vi "GetCustomDeviceTimingSourceVIs.vi"(8 "error in (no error)":errorcluster, 11 "custom device reference in":refnum<k39>) -> (0 "error out":errorcluster, 2 "timing source VIs":T1(array[cluster]), 3 "custom device reference out":refnum<k39>)   [LabVIEW 2027, in "VeriStandTestUtilities.lvlib"]
uses:
  VeriStandTestUtilities.lvlib
  C:/NetCoreDLL/NationalInstruments.VeriStand.XMLReader.dll
  NetCoreDLL/NationalInstruments.VeriStand.XMLReader.dll
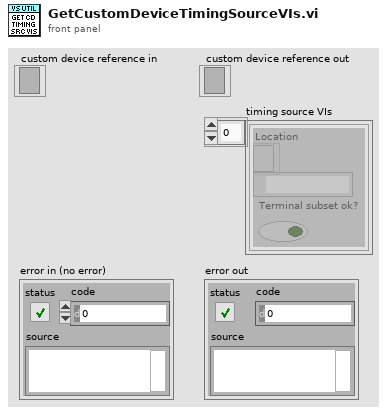
[diagram p1: front panel]
types:
  T1 = cluster{"Location":refnum<k39>, path, "Terminal subset ok?":bool}[]
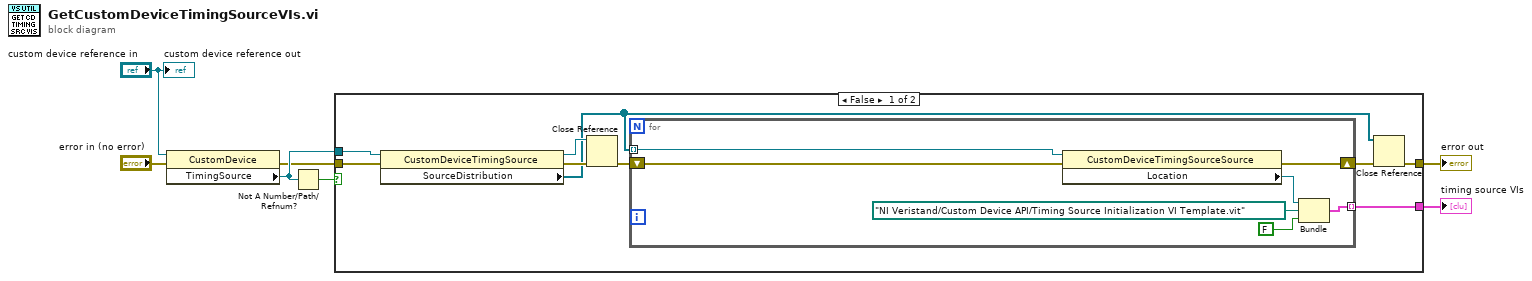
[diagram p0: block diagram]
diagram:
  n1 = property class="CustomDevice"(reference="custom device reference in", error in="error in (no error)") -> (error out=w2:errorcluster, "TimingSource"=w4:refnum<k39>)  [unwired: 1 out]
  n2 = Not A Number/Path/Refnum?(number/path/refnum=w4) -> (NaN/Path/Refnum?=w5:bool)
  n3 = case shown="False" w5 {
    tunnel: w4 -> [w16 _]
    tunnel: [w15 _] -> w7
    tunnel: w2 -> [w14 w24]
    tunnel: [w9 w24] -> w1
    frame False {
      n4 = property class="CustomDeviceTimingSource"(reference=w16, error in=w14) -> (reference out=w10:refnum<k39>, error out=w13:errorcluster, "SourceDistribution"=w8:refnum<k39>[])
      n5 = Close Reference(reference=w10, error in (no error)=w13) -> (error out=w11:errorcluster)
      n6 = for {
        tunnel: w8 -> [w23] mode=indexing
        tunnel: [w20] -> w15 mode=indexing
        shift-right: [w18] -> w12
        shift-left: w11 -> [w19]
        n7 = property class="CustomDeviceTimingSourceSource"(reference=w23, error in=w19) -> (error out=w18:errorcluster, "Location"=w22:refnum<k39>)  [unwired: 1 out]
        n8 = Bundle("Location"=w22, path "NI Veristand/Custom Device API/Timing Source Initialization VI Template.vit", FALSE) -> (w20:cluster{"Location":refnum<k39>, path, bool})  [unwired: 1 in]
      }
      n9 = Close Reference(reference=w8, error in (no error)=w12) -> (error out=w9:errorcluster)
    }
    frame True {
    }
  }
  "timing source VIs" <- w7
  "error out" <- w1
  "custom device reference out" <- "custom device reference in"
